vi "NewItem.vi"(8 "error in (no error)":errorcluster, 10 "Folder?":bool, 11 "TreeControl in":refnum<vi>) -> (0 "error out":errorcluster, 3 "TreeControl out":refnum<vi>)   [LabVIEW 2020, in "ScriptManager.lvlib"]
uses:
  ScriptManager.lvlib
  lib/UI/TreeControl/TreeControlLib.lvlib
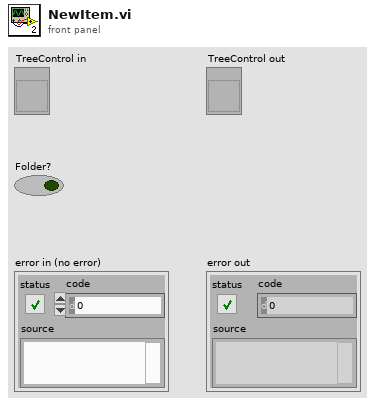
[diagram p1: front panel]
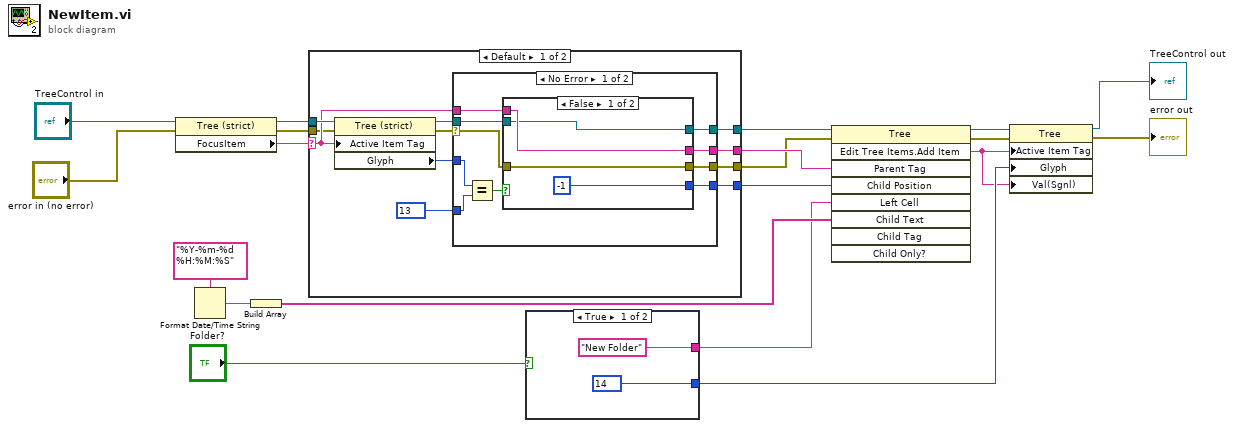
[diagram p0: block diagram]
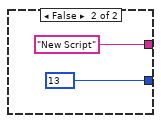
[diagram p2: hidden frame]
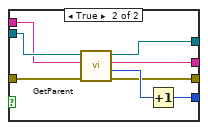
[diagram p3: hidden frame]
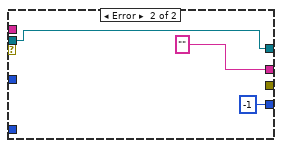
[diagram p4: hidden frame]
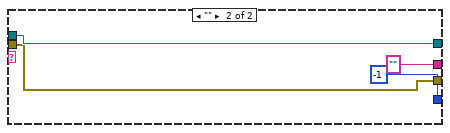
[diagram p5: hidden frame]
diagram:
  n1 = property class="Tree (strict)"(reference="TreeControl in", error in="error in (no error)") -> (reference out=w8:refnum<vi>, error out=w5:errorcluster, "FocusItem"=w17:string)
  n2 = Format Date/Time String(time format string (%c)="%Y-%m-%d %H:%M:%S") -> (date/time string=w19:string)  [unwired: 2 in]
  n3 = Build Array(w19) -> (w13:string[])
  n4 = case shown="Default" w17 {
    selector: w17 -> [w27 _]
    tunnel: w8 -> [w31 w58]
    tunnel: [w26 "" ("Parent Tag")] -> w11
    tunnel: [w25 -1 ("Child Index")] -> w10
    tunnel: [w24 w58] -> w7
    tunnel: w5 -> [w23 w57]
    tunnel: [w22 w57] -> w4
    frame Default {
      n5 = property class="Tree (strict)"(reference=w31, error in=w23, "Active Item Tag"=w27) -> (reference out=w29:refnum<vi>, error out=w21:errorcluster, "Glyph"=w30:i32)
      n6 = case shown="No Error" w21 {
        selector: w21 -> [w32 _]
        tunnel: w30 -> [w41 _]
        tunnel: w29 -> [w39 w54]
        tunnel: 13 -> [w38 _]
        tunnel: w27 -> [w37 _]
        tunnel: [w36 "" ("Parent Tag")] -> w26
        tunnel: [w35 -1 ("Child Index")] -> w25
        tunnel: [w34 w54] -> w24
        tunnel: [w33 _] -> w22
        frame No Error {
          n7 = Equal?(x=w41, y=w38) -> (x = y?=w40:bool)
          n8 = case shown="False" w40 {
            tunnel: w39 -> [w43 w53]
            tunnel: w37 -> [w45 w52]
            tunnel: [w45 w51] -> w36
            tunnel: [-1 ("Child Index") w46] -> w35
            tunnel: [w43 w49] -> w34
            tunnel: w32 -> [w42 w48]
            tunnel: [w42 w47] -> w33
            frame False {
            }
            frame True {
              n9 = call "GetParent.vi"("error in (no error)"=w48, "Tag"=w52, "TreeControl in"=w53) -> ("error out"=w47:errorcluster, "Child Index"=w50:i32, "Parent Tag"=w51:string, "TreeControl out"=w49:refnum<vi>)  [unwired: 5 in]
              n10 = Increment(x=w50) -> (x+1=w46:i32)
            }
          }
        }
        frame Error {
        }
      }
    }
    frame "" {
    }
  }
  n11 = case shown="True" "Folder?" {
    tunnel: [14 13] -> w14
    tunnel: ["New Folder" ("Left Cell String") "New Script" ("Left Cell String")] -> w12
    frame True {
    }
    frame False {
    }
  }
  n12 = invoke class="Tree" method="Edit Tree Items.Add Item"(reference=w7, error in=w4, "Parent Tag"=w11, "Child Position"=w10, "Left Cell"=w12, "Child Text"=w13) -> (reference out=w15:refnum<vi>, error out=w16:errorcluster, "Edit Tree Items:Add Item"=w1:string)  [unwired: 3 in, 6 out]
  n13 = property class="Tree"(reference=w15, error in=w16, "Active Item Tag"=w1, "Glyph"=w14, "Val(Sgnl)"=w1) -> (reference out=→"TreeControl out":refnum<vi>, error out=→"error out":errorcluster)
